vi "CSMLS - Append Continuous State.vi"(6 "Loop State (S) And Arguments":string, 8 "Append? (T)":bool=TRUE, 9 "Continous Arguments (\"\")":string, 10 "Continous State":string, 11 "States Queue":string) -> (3 "Remaining States":string)   [LabVIEW 2017, in "CSM Loop Support.lvlib"]
doc: "#### CSMLS - Append Continuous State.vi\n\nAdds a loop state.\n\n-- <b>Controls</b> --\n- <b>States Queue</b>: The entire state queue is connected to this input\n- <b>Loop State(s) and Arguments</b>: Loop states\n- <b>Continuous State</b>: Loop state name\n- <b>Continuous Arguments (\"\")</b>: Loop state arguments\n- <b>Append(T)</b>: Append or not\n\n-- <b>Indicators</b> --\n- <b>Remaining States</b>: Remaining message queue"
uses:
  CSM Loop Support.lvlib
  Communicable State Machine.lvlib
  _Shared/CSM Shared.lvlib
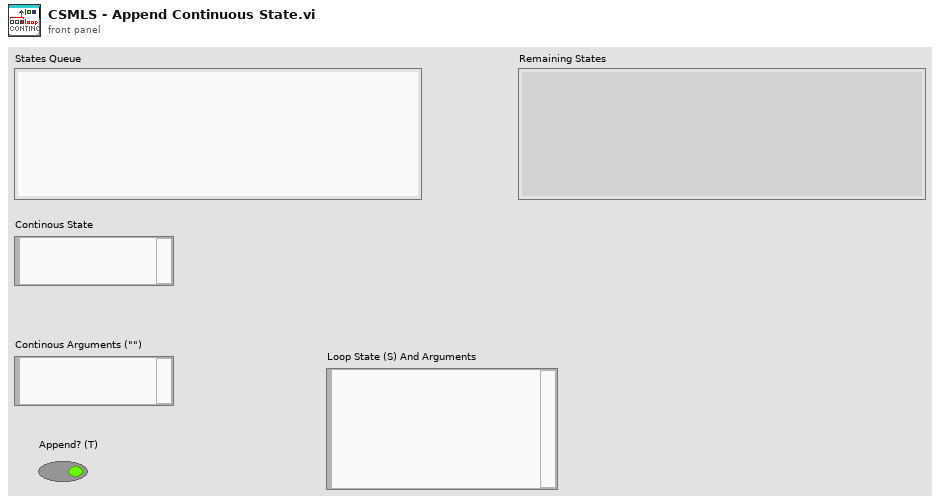
[diagram p1: front panel]
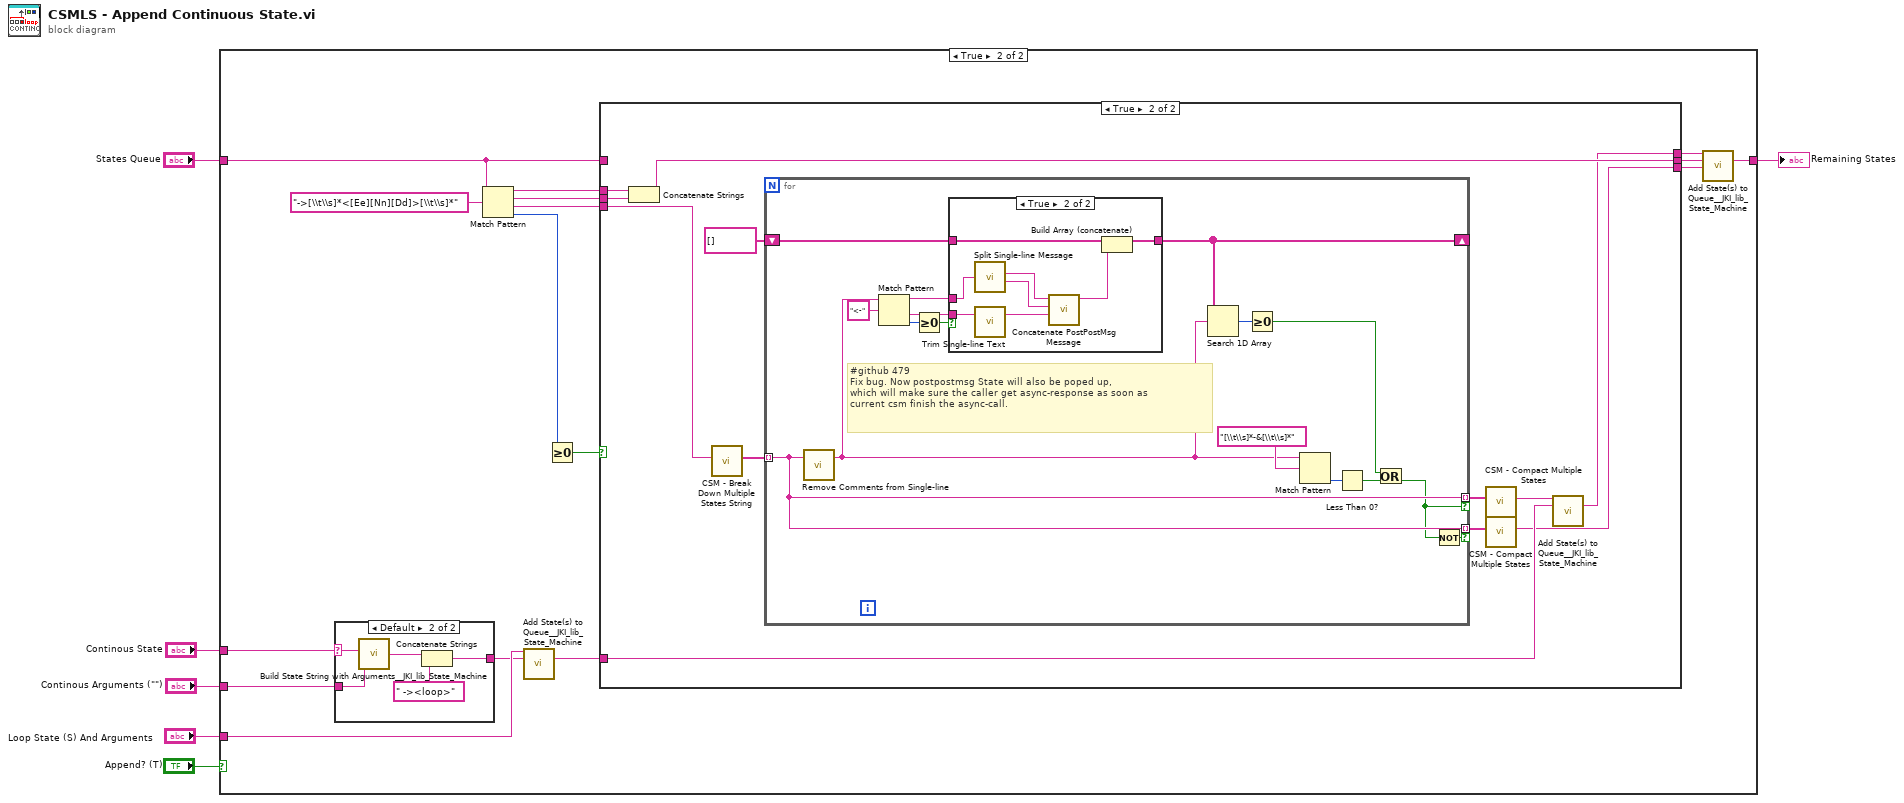
[diagram p0: block diagram]
diagram:
  n1 = case shown="True" "Append? (T)" {
    tunnel: [w7 w23] -> w6
    tunnel: "Continous Arguments (\"\")" -> [_ w22]
    tunnel: "Continous State" -> [_ w21]
    tunnel: "Loop State (S) And Arguments" -> [_ w20]
    tunnel: "States Queue" -> [w7 w14]
    frame False {
    }
    frame True {
      n2 = case shown="Default" w21 {
        selector: w21 -> [_ w27]
        tunnel: w22 -> [_ w28]
        tunnel: [_ w25] -> w19
        frame "" {
        }
        frame Default {
          n3 = call <vilib>:"Build State String with Arguments__JKI_lib_State_Machine.vi"("Arguments (\"\")"=w28, "State"=w27) -> ("State with Arguments"=w26:string)  [unwired: 4 in]
          n4 = Concatenate Strings(w26, " -><loop>" ("string")) -> (w25:string)
        }
      }
      n5 = Match Pattern(string=w14, regular expression="->[\\t\\s]*<[Ee][Nn][Dd]>[\\t\\s]*") -> (before substring=w13:string, match substring=w12:string, after substring=w11:string, offset past match=w17:i32)  [unwired: 1 in]
      n6 = call <vilib>:"Add State(s) to Queue__JKI_lib_State_Machine.vi"("State(s) in Front (\"\")"=w20, "State(s) in (\"\")"=w19) -> ("States Out"=w9:string)  [unwired: 13 in]
      n7 = Greater Or Equal To 0?(x=w17) -> (x >= 0?=w16:bool)
      n8 = case shown="True" w16 {
        tunnel: [w30 w40] -> w15
        tunnel: w14 -> [w30 _]
        tunnel: w13 -> [_ w42]
        tunnel: w12 -> [_ w41]
        tunnel: w11 -> [_ w37]
        tunnel: [w29 w38] -> w10
        tunnel: w9 -> [w29 w39]
        tunnel: [_ w32] -> w8
        frame False {
        }
        frame True {
          n9 = Concatenate Strings(w42, w41) -> (w40:string)
          n10 = call "CSM - Break Down Multiple States String.vi"("States"=w37) -> ("Multiple States"=w36:string[])  [unwired: 10 in]
          n11 = for {
            tunnel: w36 -> [w56] mode=indexing
            tunnel: [w56] -> w34 mode=indexing if=w45
            tunnel: [w56] -> w35 mode=indexing if=w54
            shift-right: [w47] -> _
            shift-left: string[] [] ("PostPostMsg Message") -> [w48]
            # "#github 479\nFix bug. Now postpostmsg State will also be poped up,\nwhich will make sure the caller get async-response as soon as\ncurrent csm finish the async-call."
            n12 = call "Remove Comments from Single-line.vi"("single-line text"=w56) -> ("single-line text without comments"=w46:string)  [unwired: 2 in]
            n13 = Match Pattern(string=w46, regular expression="<-") -> (before substring=w49:string, after substring=w50:string, offset past match=w52:i32)  [unwired: 1 in, 1 out]
            n14 = Greater Or Equal To 0?(x=w52) -> (x >= 0?=w51:bool)
            n15 = case shown="True" w51 {
              tunnel: w50 -> [_ w67]
              tunnel: w49 -> [_ w66]
              tunnel: [w59 w61] -> w47
              tunnel: w48 -> [w59 w62]
              frame False {
              }
              frame True {
                n16 = call "Split Single-line Message.vi"("single-line text"=w66) -> ("state"=w65:string, "args"=w64:string)  [unwired: 6 in, 2 out]
                n17 = call "Trim Single-line Text.vi"("single-line text"=w67) -> ("trimed text"=w63:string)  [unwired: 2 in]
                n18 = call "Concatenate PostPostMsg Message.vi"("Source"=w63, "Arguments"=w64, "Async-Message"=w65) -> ("PostPostMsg Message"=w60:string)  [unwired: 8 in]
                n19 = Build Array (concatenate)(w62, w60) -> (w61:string[])
              }
            }
            n20 = Search 1D Array(1D array=w47, element=w46) -> (index of element=w44:i32)  [unwired: 1 in]
            n21 = Greater Or Equal To 0?(x=w44) -> (x >= 0?=w43:bool)
            n22 = Match Pattern(string=w46, regular expression="[\\t\\s]*-&[\\t\\s]*") -> (offset past match=w57:i32)  [unwired: 1 in, 3 out]
            n23 = Less Than 0?(x=w57) -> (x < 0?=w55:bool)
            n24 = Or(x=w43, y=w55) -> (x .or. y?=w45:bool)
            n25 = Not(x=w45) -> (.not. x?=w54:bool)
          }
          n26 = call "CSM - Compact Multiple States.vi"("Multiple States"=w34) -> ("States"=w33:string)  [unwired: 9 in]
          n27 = call "CSM - Compact Multiple States.vi"("Multiple States"=w35) -> ("States"=w32:string)  [unwired: 9 in]
          n28 = call <vilib>:"Add State(s) to Queue__JKI_lib_State_Machine.vi"("State(s) in Front (\"\")"=w33, "State(s) in (\"\")"=w39) -> ("States Out"=w38:string)  [unwired: 13 in]
        }
      }
      n29 = call <vilib>:"Add State(s) to Queue__JKI_lib_State_Machine.vi"("State(s) in Front (\"\")"=w10, "State(s) in (\"\")"=w15, "State(s) at Back (\"\")"=w8) -> ("States Out"=w23:string)  [unwired: 12 in]
    }
  }
  "Remaining States" <- w6
